vi "tm_getnextframe_a.vi"(7 "Timeout":i32=-1, 8 "error in (no error)":errorcluster, 10 "Buffer":u16[][](array[numeric]), 11 "Handle in":u32) -> (0 "error out":errorcluster, 2 "Data":u16[][](array[numeric]), 3 "Handle out":u32)   [LabVIEW 2017]
uses:
  tmcamcon.dll
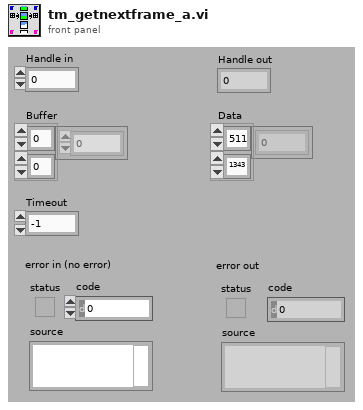
[diagram p1: front panel]
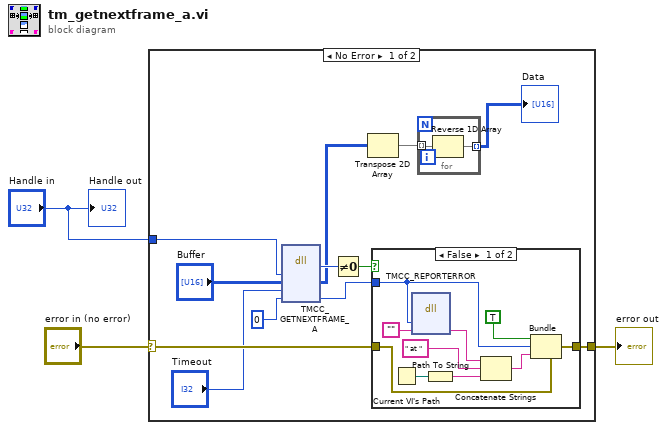
[diagram p0: block diagram]
diagram:
  n1 = case shown="No Error" "error in (no error)" {
    selector: "error in (no error)" -> [w10 w29]
    tunnel: [w9 w29] -> w2
    tunnel: "Handle in" -> [w8 _]
    frame No Error {
      n2 = dll-call lib="tmcamcon.dll" fn="TMCC_GETNEXTFRAME_A"("index"=w8, "imgarray"="Buffer", "timeout"="Timeout", "Erval"=0) -> ("return type"=w15:u32, "imgarray"=w4:u16[][], "Erval"=w11:i32)  [unwired: 5 in, 2 out]
      n3 = Not Equal To 0?(x=w15) -> (x != 0?=w12:bool)
      n4 = Transpose 2D Array(2D array=w4) -> (transposed array=w6:u16[][])
      n5 = case shown="False" w12 {
        tunnel: w10 -> [w27 w28]
        tunnel: [w26 w28] -> w9
        tunnel: w11 -> [w20 _]
        frame False {
          n6 = Current VI's Path() -> (path=w25:path)
          n7 = dll-call lib="tmcamcon.dll" fn="TMCC_REPORTERROR"("error"=w20, "buf"="") -> ("buf"=w19:string)  [unwired: 5 in, 2 out]
          n8 = Path To String(path=w25) -> (string=w21:string)
          n9 = Concatenate Strings(w19, " at ", w21) -> (w24:string)
          n10 = Bundle(cluster=w27, "status"=TRUE, "code"=w20, "source"=w24) -> (w26:errorcluster)
        }
        frame True {
        }
      }
      n11 = for {
        tunnel: w6 -> [w17] mode=indexing
        tunnel: [w16] -> w5 mode=indexing
        n12 = Reverse 1D Array(array=w17) -> (reversed array=w16:u16[])
      }
      "Data" <- w5
    }
    frame Error {
    }
  }
  "error out" <- w2
  "Handle out" <- "Handle in"
